vi "Test RoundTrip Path.vi"(8 "error in (no error)":errorcluster) -> (0 "error out":errorcluster)   [LabVIEW 2013]
uses:
  <vilib>/addons/_JKI Toolkits/Caraya/classes/Test/Test.lvclass
  <vilib>/addons/_JKI Toolkits/Caraya/classes/Assert/Assert.lvclass
  src/JKI JSON Serialization.lvlib
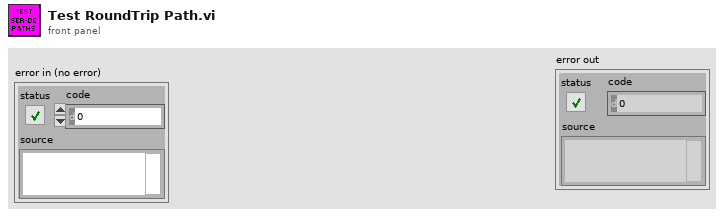
[diagram p1: front panel]
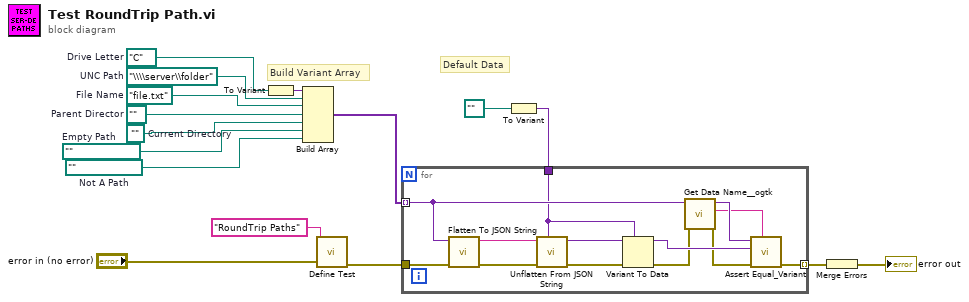
[diagram p0: block diagram]
diagram:
  w4 = path ""  # Not A Path
  w11 = path "file.txt"  # File Name
  w12 = path "\\\\server\\folder"  # UNC Path
  w3 = path "C:/"  # Drive Letter
  w8 = path ""  # Empty Path
  w9 = path ""  # Current Directory
  w10 = path ".."  # Parent Director
  # "Build Variant Array"
  # "Default Data"
  n1 = To Variant(anything=w3) -> (Variant=w1:variant)
  n2 = Build Array(w1, w12, w11, w10, w9, w8, w4) -> (w2:variant[])
  n3 = call <vilib>:"Define Test.vi"("error in (no error)"="error in (no error)", "Label (VI Title)"="RoundTrip Paths") -> ("error out"=w5:errorcluster)  [unwired: 9 in]
  n4 = To Variant(anything=path "") -> (Variant=w6:variant)
  n5 = for {
    tunnel: w2 -> [w25] mode=indexing
    tunnel: w5 -> [w20]
    tunnel: [w19] -> w14 mode=indexing
    tunnel: w6 -> [w18]
    n6 = call "Flatten To JSON String.vi"("error in (no error)"=w20, "Variant"=w25) -> ("error out"=w29:errorcluster, "JSON String"=w17:string)  [unwired: 8 in]
    n7 = call "Unflatten From JSON String.vi"("Type and Defaults"=w18, "error in (no error)"=w29, "JSON String"=w17) -> ("error out"=w26:errorcluster, "Variant"=w28:variant)  [unwired: 7 in]
    n8 = Variant To Data(error in=w26, type=w18, Variant=w28) -> (data=w27:variant, error out=w22:errorcluster)
    n9 = call <userlib>:"Get Data Name__ogtk.vi"("error in (no error)"=w22, "Data"=w25) -> ("error out"=w21:errorcluster, "Data Name"=w23:string, "Data dup"=w24:variant)  [unwired: 7 in]
    n10 = call <vilib>:"Assert Equal_Variant.vi"("Label"=w23, "error in (no error)"=w21, "Y"=w27, "X"=w24) -> ("error out"=w19:errorcluster)  [unwired: 7 in]
  }
  n11 = Merge Errors(w14) -> (→"error out":errorcluster)
